vi "manageQueue.vi"(6 "MessageQRef":refnum<queue>, 8 "error in (no error)":errorcluster, 9 "FNs":enum16{"Back", "Front", "Replace"}(ring), 10 "Message":T1(array[cluster]), 11 "CameraNetworkClient in":refnum<class "CameraNetworkServer.lvclass">) -> (0 "error out":errorcluster, 3 "CameraNetworkClient out":refnum<class "CameraNetworkServer.lvclass">)   [LabVIEW 2011, in "Hardware.lvlib" / "HWControllers.lvlib" / "CameraNetworkServer.lvclass"]
uses:
  CameraNetworkServer.lvclass
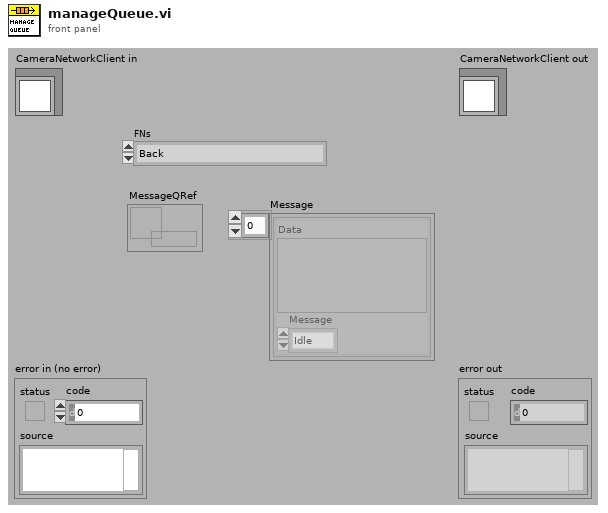
[diagram p1: front panel]
types:
  T1 = cluster{"Message":enum16{"Idle", "initialise", "configureAcquisition", "setTemperature", "getTemperature", "start", "stop", "sendImage", "close", "error", "ExitApp", "getAcquisitionStatus"}, "Data":variant}[]
  T2 = cluster{"Message":enum16{"Idle", "initialise", "configureAcquisition", "setTemperature", "getTemperature", "start", "stop", "sendImage", "close", "error", "ExitApp"}, "Data":variant}
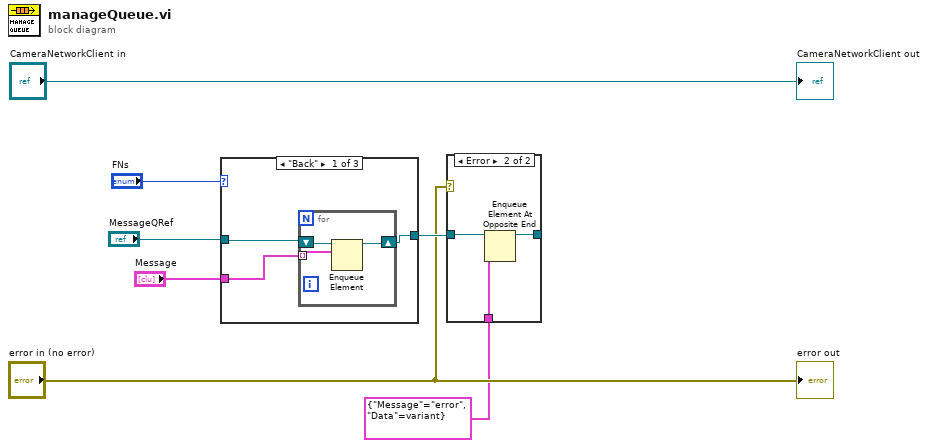
[diagram p0: block diagram]
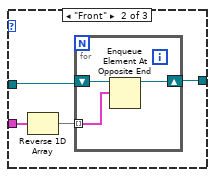
[diagram p3: hidden frame]
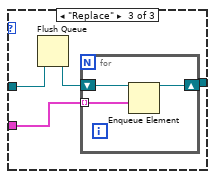
[diagram p4: hidden frame]
diagram:
  n1 = case shown="\"Back\"" "FNs" {
    tunnel: "Message" -> [w8 w17 w22]
    tunnel: "MessageQRef" -> [w10 w15 w24]
    tunnel: [w9 w14 w21] -> w6
    frame "Back" {
      n2 = for {
        shift-right: [w12] -> w9
        shift-left: w10 -> [w13]
        tunnel: w8 -> [w11] mode=indexing
        n3 = Enqueue Element(queue=w13, element=w11) -> (queue out=w12:refnum<queue>)  [unwired: 2 in, 2 out]
      }
    }
    frame "Front" {
      n4 = Reverse 1D Array(array=w17) -> (reversed array=w16:T1)
      n5 = for {
        tunnel: w16 -> [w19] mode=indexing
        shift-right: [w18] -> w14
        shift-left: w15 -> [w20]
        n6 = Enqueue Element At Opposite End(queue=w20, element=w19) -> (queue out=w18:refnum<queue>)  [unwired: 2 in, 2 out]
      }
    }
    frame "Replace" {
      n7 = Flush Queue(queue=w24) -> (queue out=w23:refnum<queue>)  [unwired: 1 in, 2 out]
      n8 = for {
        tunnel: w22 -> [w26] mode=indexing
        shift-right: [w25] -> w21
        shift-left: w23 -> [w27]
        n9 = Enqueue Element(queue=w27, element=w26) -> (queue out=w25:refnum<queue>)  [unwired: 2 in, 2 out]
      }
    }
  }
  n10 = case shown="Error" "error in (no error)" {
    tunnel: w6 -> [w28 w31]
    tunnel: [w28 w30] -> _
    tunnel: T2 {"Message"=enum."error", "Data"=variant} -> [_ w29]
    frame No Error {
    }
    frame Error {
      n11 = Enqueue Element At Opposite End(queue=w31, element=w29) -> (queue out=w30:refnum<queue>)  [unwired: 2 in, 2 out]
    }
  }
  "error out" <- "error in (no error)"
  "CameraNetworkClient out" <- "CameraNetworkClient in"
